vi "Backup or Restore GFG Config Data.vi"(7 "Action Select":T1, 8 "error in (no error)":errorcluster) -> (0 "error out":errorcluster)   [LabVIEW 2012]
doc: "SciScan 1.2 160622"
uses:
  Backup or Restore GFG Config Data_Commands.ctl
  MacroGUI Module/SubVIs/MacroFileIO_Commands.ctl
  INI/settingsIO/Settings IO_Commands.ctl
  MacroGUI Module/Custom Controls and Typedefs/GFG Variable for IO.ctl
panel:
  out "Array":string[](array[string])
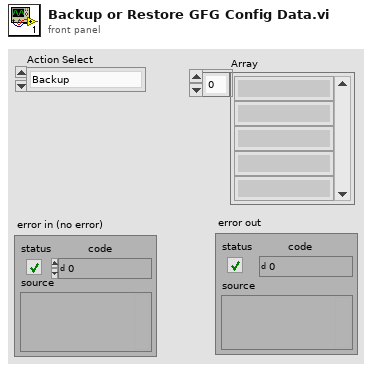
[diagram p1: front panel]
types:
  T1 = typedef "Backup or Restore GFG Config Data_Commands.ctl" = enum16{"Backup", "Restore"}
  T2 = typedef "MacroFileIO_Commands.ctl" = enum16{"Get Macro Info", "Initialize", "New Macro", "Load Macro", "Save", "Save in today's folder", "Update Settings File", "Add Settings File", "Delete Settings File", "Update Macro Text", "Save As", "Read Temp File"}
  T3 = typedef "Settings IO_Commands.ctl" = enum16{"Write HW Settings", "Write Config Settings", "Read HW Settings", "Read Config Settings", "Write Line-Scan Settings", "Write Frame-Scan Settings", "Write Z-Stack Settings", "Read Line-Scan Settings", "Read Frame-Scan Settings", "Read Z-Stack Settings", "Read Fast-Z Settings", "Write Fast-Z Settings"}
  T4 = enum16{"Get Settings Table ", "Read Settings File", "Get Specified Settings"}
  T5 = typedef "GFG Variable for IO.ctl" = cluster{"Variable Name":string, "Value (Variant)":variant, "data type":string}
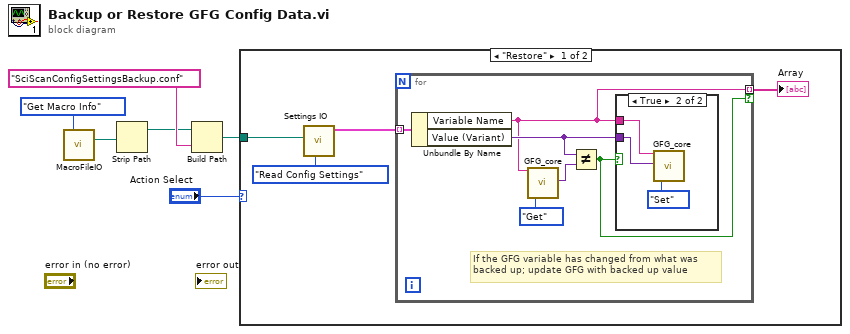
[diagram p0: block diagram]
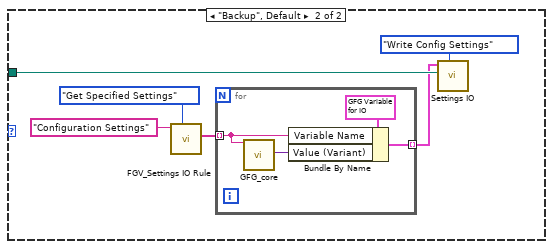
[diagram p3: hidden frame]
diagram:
  n1 = call "MacroFileIO.vi"("MacroFileIO_Command"=MacroFileIO_Commands."Get Macro Info") -> ("Temp File path"=w2:path)  [unwired: 9 in, 5 out]
  n2 = Strip Path(path=w2) -> (stripped path=w4:path)  [unwired: 1 out]
  n3 = Build Path(base path=w4, name or relative path="SciScanConfigSettingsBackup.conf") -> (appended path=w6:path)
  n4 = case shown="\"Restore\"" "Action Select" {
    tunnel: w6 -> [w9 w25]
    frame "Restore" {
      n5 = call "Settings IO.vi"("SettingsFileIO_Commands"=Settings_IO_Commands."Read Config Settings", "File Path (for scan specific settings)"=w9) -> ("Settings Array OUT"=w8:T5[])  [unwired: 7 in, 2 out]
      n6 = for {
        tunnel: w8 -> [w16] mode=indexing
        tunnel: [w12] -> w7 mode=indexing if=w11
        # "If the GFG variable has changed from what was\nbacked up; update GFG with backed up value"
        n7 = Unbundle By Name(w16) -> ("Variable Name"=w12:string, "Value (Variant)"=w13:variant)
        n8 = call "GFG_core.vi"("Variable Name in"=w12, "Action"=enum16{"Init", "Set", "Get", "Clear"}."Get") -> ("Variant Out"=w14:variant)  [unwired: 11 in, 6 out]
        n9 = Not Equal?(x=w13, y=w14) -> (x != y?=w11:bool)
        n10 = case shown="True" w11 {
          tunnel: w13 -> [_ w17]
          tunnel: w12 -> [_ w18]
          frame False {
          }
          frame True {
            n11 = call "GFG_core.vi"("Variable Name in"=w18, "Variant in"=w17, "Action"=enum16{"Init", "Set", "Get", "Clear"}."Set") -> ()  [unwired: 10 in, 7 out]
          }
        }
      }
      "Array" <- w7
    }
    frame "Backup", Default {
      n12 = call "FGV_Settings IO Rule.vi"("Command_Settings IO Rule"=T4."Get Specified Settings", "Settings Type IN"="Configuration Settings") -> ("Specified Settings (OUT)"=w23:string[])  [unwired: 7 in, 2 out]
      n13 = for {
        tunnel: w23 -> [w27] mode=indexing
        tunnel: [w26] -> w24 mode=indexing
        n14 = call "GFG_core.vi"("Variable Name in"=w27) -> ("Variant Out"=w28:variant)  [unwired: 12 in, 6 out]
        n15 = Bundle By Name(cluster=T5 {"Variable Name"="", "Value (Variant)"=variant, "data type"=""}, "Variable Name"=w27, "Value (Variant)"=w28) -> (w26:T5)
      }
      n16 = call "Settings IO.vi"("SettingsFileIO_Commands"=Settings_IO_Commands."Write Config Settings", "File Path (for scan specific settings)"=w25, "Settings Array IN"=w24) -> ()  [unwired: 6 in, 3 out]
    }
  }
